vi "CDEx Redesign Controller for 3DoF Helicopter OnTheFly.vi"() -> ()   [LabVIEW 2009]
doc: "This example is derived from the Quanser (www.quanser.com) 3 DOF Helicopter academic challenge."
uses:
  <vilib>/addons/Control Design/_Model Construction/Model Creation.llb/Model Creation SubVI/cd_Create Symbolic State Space Model.vi
  <vilib>/Analysis/7linalg.llb/Create Special Real Matrix.vi
  3DHe_Global.vi
  <vilib>/addons/Control Design/_State Feedback Control/State Feedback Control.llb/State Feedback Control SubVis/cd_Linear Quadratic Regulator.vi
  <vilib>/Analysis/Matrix/Numeric/Conversions/Matrix To Array - RM.vi
  <vilib>/Analysis/NI_AALPro.lvlib
  <vilib>/addons/Control Design/_Model Construction/NI_LinSys_Model Creation.lvlib
  <vilib>/addons/Control Design/_State Feedback Control/NI_CD_State Feedback Control.lvlib
  <vilib>/Analysis/Matrix/NI_Matrix.lvlib
panel:
  in  "End":bool
  out "Tab Control":enum32{"Control Design: LQR"}(tab)
  in  "Diagonal of Q":dbl[](array[numeric])=[100.0, 100.0, 4000.0, 60.0, 100.0, 1500.0, 50.0, 10.0] format="%#.2g"
  out "Kep [V/deg]":dbl=-0.1888101782609241 format="%.2f"
  out "Ked [V/ deg sec^-1]":dbl=-0.148727007678325 format="%.2f"
  out "Kei [V/deg sec]":dbl=-0.07845852415328128 format="%.2f"
  out "Kpp [V/deg]":dbl=-0.40085841198215855 format="%.2f"
  out "Kpd [V/deg sec^-1]":dbl=-0.130295098559931 format="%.2f"
  out "Kpi":dbl format="%.2f"
  out "Ktp [deg/deg]":dbl=1.8918979439912578 format="%.2f"
  out "Ktd [deg/deg sec^-1]":dbl=2.9393753016474626 format="%.2f"
  out "Kti [deg/deg sec]":dbl=0.08753147368150993 format="%.2f"
  out "Optimal Gain (K)":dbl[][](array[numeric])=[[5.3810900382573665, 11.424464804866695, -21.613921777920005, 4.238719740944304, 3.7134103122560975, -33.580789896433664, 2.2360680469486356, -1.0000002670378931], [5.3810901226153085, -11.424464678116344, 21.613920933336832, 4.238719696720222, -3.71341030565997, 33.580789094931205, 2.2360678297883974, 1.000000202652513]] format="%.2f"
  in  "Design Method":u16(ring)=2 items=["manual", "stiff in elevation", "stiff in travel", "stiff in pitch", "minimize control"]
  in  "R":dbl[][](array[numeric])=[[5.0, 0.0], [0.0, 5.0]] format="%#.2g"
  in  "Q":dbl[][](array[numeric])=[[100.0, 0.0, 0.0, 0.0, 0.0, 0.0, 0.0, 0.0], [0.0, 100.0, 0.0, 0.0, 0.0, 0.0, 0.0, 0.0], [0.0, 0.0, 4000.0, 0.0, 0.0, 0.0, 0.0, 0.0], [0.0, 0.0, 0.0, 60.0, 0.0, 0.0, 0.0, 0.0], [0.0, 0.0, 0.0, 0.0, 100.0, 0.0, 0.0, 0.0], [0.0, 0.0, 0.0, 0.0, 0.0, 1500.0, 0.0, 0.0], [0.0, 0.0, 0.0, 0.0, 0.0, 0.0, 50.0, 0.0], [0.0, 0.0, 0.0, 0.0, 0.0, 0.0, 0.0, 10.0]] format="%#.2g"
  # "Derived Control Parameters\nfor PID Controllers from\nOptimal Gain"
  # "Control Design: LQR"
  # "Change the Design Method or the values in the Q and R matrices to verify the response in Simulation."
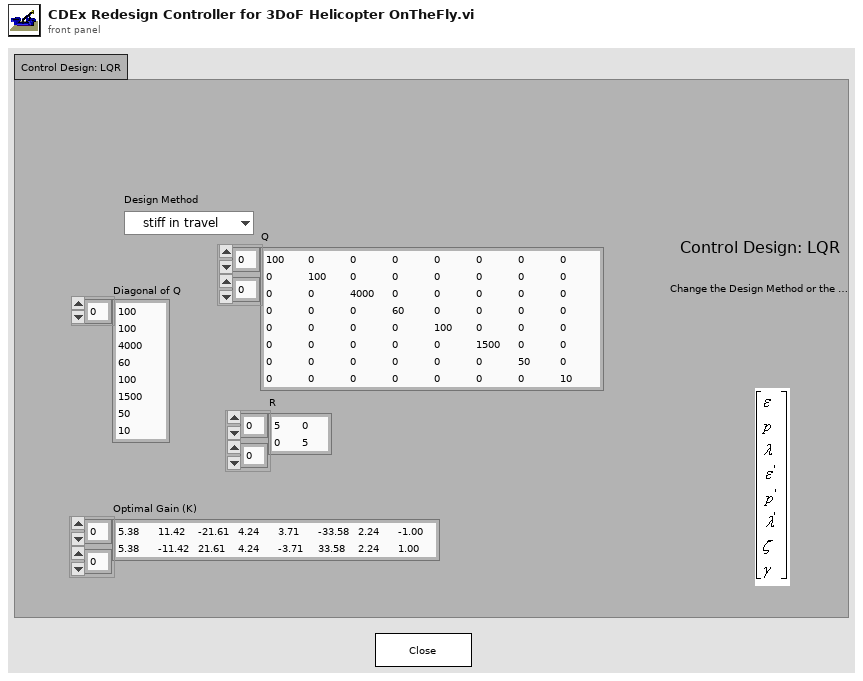
[diagram p1: front panel]
types:
  T1 = enum32{"Identity", "Diagonal", "Toepliz", "Vandermonde", "Companion"}
  T2 = typedef "NI_Matrix.lvlib/RealMatrix.ctl" = dbl[][]
  T3 = typedef "NI_LinSys_Model Typedefs.lvlib/CD State Space Model (MIMO).ctl" = cluster{"properties":T4, "A":dbl[][], "B":dbl[][], "C":dbl[][], "D":dbl[][], "StateNames":string[], "Transport Delay":dbl[][]}
  T4 = typedef "NI_LinSys_Model Typedefs.lvlib/CD General Elements.ctl" = cluster{"Model name":string, "Input names":string[], "Output names":string[], "Input Delays":dbl[], "Output Delays":dbl[], "Sampling Time":dbl, "Notes":string}
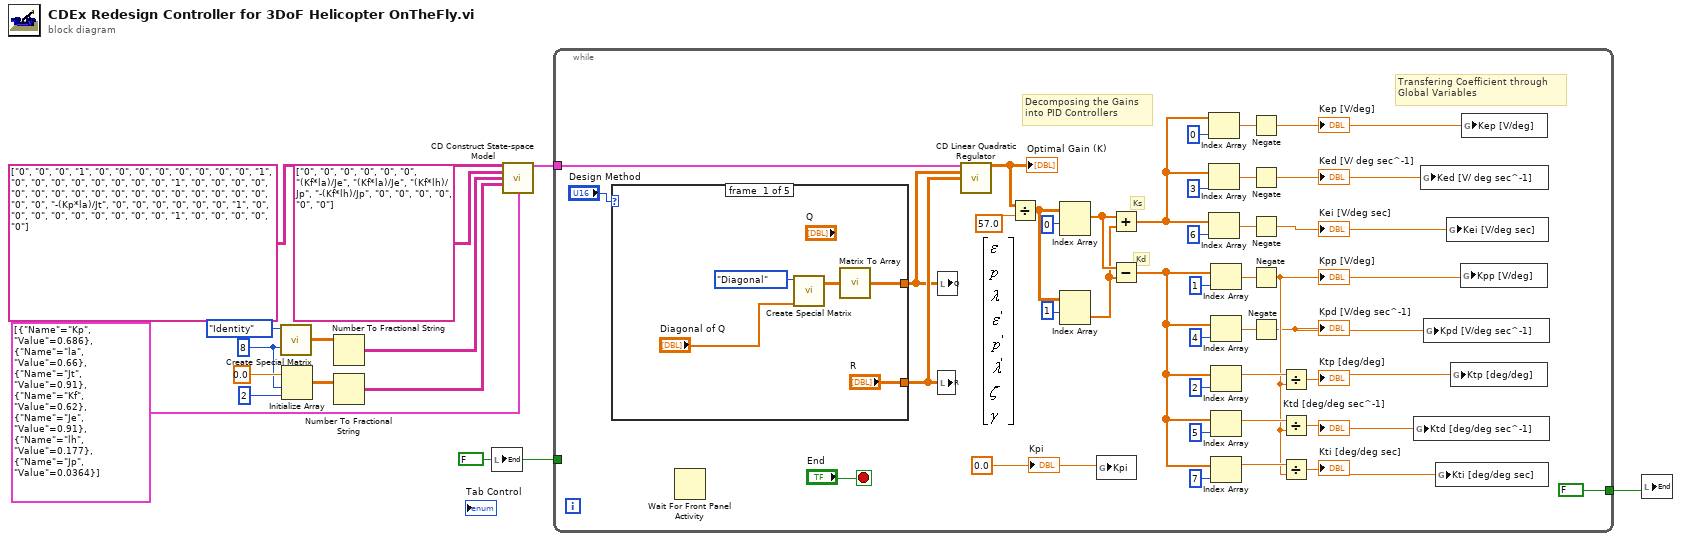
[diagram p0: block diagram]
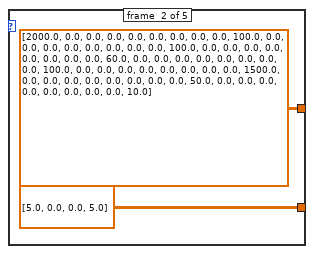
[diagram p2: hidden frame]
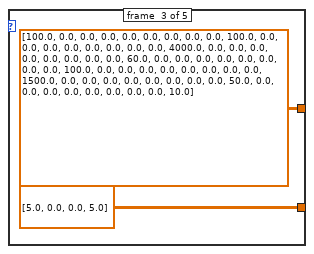
[diagram p3: hidden frame]
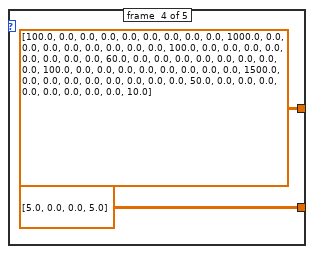
[diagram p4: hidden frame]
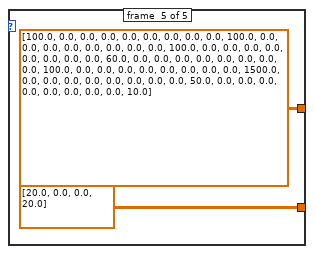
[diagram p5: hidden frame]
diagram:
  w2 = FALSE ("End")
  w9 = 8 ("matrix size")
  n1 = call-poly <vilib>:"Create Special Matrix.vi"("matrix type"=T1."Identity", "matrix size"=w9) -> ("Special Matrix"=w8:T2)  [unwired: 2 in, 2 out]
  n2 = Initialize Array(0.0 ("element"), w9, 2 ("dimension size")) -> (w12:dbl[][])
  n3 = Number To Fractional String(number=w8) -> (F-format string=w14:string[][])  [unwired: 3 out]
  n4 = Number To Fractional String(number=w12) -> (F-format string=w13:string[][])  [unwired: 3 out]
  n5 = local write "End"(w2) -> ()
  n6 = call-poly <vilib>:"CD Construct State-space Model.vi"("Symbolic A"=string[][] [["0", "0", "0", "1", "0", "0", "0", "0"], ["0", "0", "0", "0", "1", "0", "0", "0"], ["0", "0", "0", "0", "0", "1", "0", "0"], ["0", "0", "0", "0", "0", "0", "0", "0"], ["0", "0", "0", "0", "0", "0", "0", "0"], ["0", "-(Kp*la)/Jt", "0", "0", "0", "0", "0", "0"], ["1", "0", "0", "0", "0", "0", "0", "0"], ["0", "0", "1", "0", "0", "0", "0", "0"]] ("A"), "Symbolic B"=string[][] [["0", "0"], ["0", "0"], ["0", "0"], ["(Kf*la)/Je", "(Kf*la)/Je"], ["(Kf*lh)/Jp", "-(Kf*lh)/Jp"], ["0", "0"], ["0", "0"], ["0", "0"]] ("B"), "Symbolic C"=w14, "Symbolic D"=w13, "Variables"=cluster{"Name":string, "Value":dbl}[] [{"Name"="Kp", "Value"=0.686}, {"Name"="la", "Value"=0.66}, {"Name"="Jt", "Value"=0.91}, {"Name"="Kf", "Value"=0.62}, {"Name"="Je", "Value"=0.91}, {"Name"="lh", "Value"=0.177}, {"Name"="Jp", "Value"=0.0364}]) -> ("State Space Model"=w3:T3)  [unwired: 2 in, 8 out]
  n7 = while {
    tunnel: w3 -> [w54]
    tunnel: w2 -> [_]
    tunnel: [FALSE ("End")] -> w1
    stop <- "End" stop-if-true
    w26 = 0.0
    # "Transfering Coefficient through\nGlobal Variables"
    # "Decomposing the Gains\ninto PID Controllers"
    # "Kd"
    # "Ks"
    n8 = case shown="1" "Design Method" {
      tunnel: [w55 dbl[][] [[2000.0, 0.0, 0.0, 0.0, 0.0, 0.0, 0.0, 0.0], [0.0, 100.0, 0.0, 0.0, 0.0, 0.0, 0.0, 0.0], [0.0, 0.0, 100.0, 0.0, 0.0, 0.0, 0.0, 0.0], [0.0, 0.0, 0.0, 60.0, 0.0, 0.0, 0.0, 0.0], [0.0, 0.0, 0.0, 0.0, 100.0, 0.0, 0.0, 0.0], [0.0, 0.0, 0.0, 0.0, 0.0, 1500.0, 0.0, 0.0], [0.0, 0.0, 0.0, 0.0, 0.0, 0.0, 50.0, 0.0], [0.0, 0.0, 0.0, 0.0, 0.0, 0.0, 0.0, 10.0]] ("Q") dbl[][] [[100.0, 0.0, 0.0, 0.0, 0.0, 0.0, 0.0, 0.0], [0.0, 100.0, 0.0, 0.0, 0.0, 0.0, 0.0, 0.0], [0.0, 0.0, 4000.0, 0.0, 0.0, 0.0, 0.0, 0.0], [0.0, 0.0, 0.0, 60.0, 0.0, 0.0, 0.0, 0.0], [0.0, 0.0, 0.0, 0.0, 100.0, 0.0, 0.0, 0.0], [0.0, 0.0, 0.0, 0.0, 0.0, 1500.0, 0.0, 0.0], [0.0, 0.0, 0.0, 0.0, 0.0, 0.0, 50.0, 0.0], [0.0, 0.0, 0.0, 0.0, 0.0, 0.0, 0.0, 10.0]] ("Q") dbl[][] [[100.0, 0.0, 0.0, 0.0, 0.0, 0.0, 0.0, 0.0], [0.0, 1000.0, 0.0, 0.0, 0.0, 0.0, 0.0, 0.0], [0.0, 0.0, 100.0, 0.0, 0.0, 0.0, 0.0, 0.0], [0.0, 0.0, 0.0, 60.0, 0.0, 0.0, 0.0, 0.0], [0.0, 0.0, 0.0, 0.0, 100.0, 0.0, 0.0, 0.0], [0.0, 0.0, 0.0, 0.0, 0.0, 1500.0, 0.0, 0.0], [0.0, 0.0, 0.0, 0.0, 0.0, 0.0, 50.0, 0.0], [0.0, 0.0, 0.0, 0.0, 0.0, 0.0, 0.0, 10.0]] ("Q") dbl[][] [[100.0, 0.0, 0.0, 0.0, 0.0, 0.0, 0.0, 0.0], [0.0, 100.0, 0.0, 0.0, 0.0, 0.0, 0.0, 0.0], [0.0, 0.0, 100.0, 0.0, 0.0, 0.0, 0.0, 0.0], [0.0, 0.0, 0.0, 60.0, 0.0, 0.0, 0.0, 0.0], [0.0, 0.0, 0.0, 0.0, 100.0, 0.0, 0.0, 0.0], [0.0, 0.0, 0.0, 0.0, 0.0, 1500.0, 0.0, 0.0], [0.0, 0.0, 0.0, 0.0, 0.0, 0.0, 50.0, 0.0], [0.0, 0.0, 0.0, 0.0, 0.0, 0.0, 0.0, 10.0]] ("Q")] -> w27
      tunnel: ["R" dbl[][] [[5.0, 0.0], [0.0, 5.0]] ("R") dbl[][] [[5.0, 0.0], [0.0, 5.0]] ("R") dbl[][] [[5.0, 0.0], [0.0, 5.0]] ("R") dbl[][] [[20.0, 0.0], [0.0, 20.0]] ("R")] -> w28
      frame #0 {
        n9 = call-poly <vilib>:"Create Special Matrix.vi"("matrix type"=T1."Diagonal", "Input Vector1"="Diagonal of Q") -> ("Special Matrix"=w56:T2)  [unwired: 2 in, 2 out]
        n10 = call-poly <vilib>:"Matrix To Array.vi"("Real Matrix"=w56) -> ("Real 2D Array"=w55:dbl[][])
      }
      frame #1 {
      }
      frame #2 {
      }
      frame #3 {
      }
      frame #4 {
      }
    }
    n11 = Wait For Front Panel Activity() -> ()  [unwired: 4 out]
    n12 = local write "Q"(w27) -> ()
    n13 = local write "R"(w28) -> ()
    n14 = call-poly <vilib>:"CD Linear Quadratic Regulator.vi"("State-Space Model"=w54, "Q"=w27, "R"=w28) -> ("Optimal Gain (K)"=w17:dbl[][])  [unwired: 3 in, 9 out]
    "Optimal Gain (K)" <- w17
    n15 = Divide(x=w17, y=57.0) -> (x/y=w52:dbl[][])
    n16 = Index Array(array=w52, index (row)=0 ("disabled index (col)")) -> (element=w51:dbl[])  [unwired: 1 in]
    n17 = Index Array(array=w52, index (row)=1 ("disabled index (col)")) -> (element=w50:dbl[])  [unwired: 1 in]
    n18 = global write "3DHe_Global.vi" "Kpi"(w26) -> ()
    n19 = Add(x=w51, y=w50) -> (x+y=w41:dbl[])
    n20 = Subtract(x=w51, y=w50) -> (x-y=w33:dbl[])
    n21 = Index Array(array=w41, index=0) -> (element=w48:dbl)
    n22 = Index Array(array=w41, index=3) -> (element=w46:dbl)
    n23 = Index Array(array=w41, index=6) -> (element=w43:dbl)
    n24 = Index Array(array=w33, index=1) -> (element=w38:dbl)
    n25 = Index Array(array=w33, index=4) -> (element=w39:dbl)
    n26 = Index Array(array=w33, index=2) -> (element=w32:dbl)
    n27 = Index Array(array=w33, index=5) -> (element=w31:dbl)
    n28 = Index Array(array=w33, index=7) -> (element=w30:dbl)
    n29 = Negate(x=w48) -> (-x=w25:dbl)
    "Kep [V/deg]" <- w25
    n30 = Negate(x=w46) -> (-x=w24:dbl)
    "Ked [V/ deg sec^-1]" <- w24
    n31 = Negate(x=w43) -> (-x=w23:dbl)
    "Kei [V/deg sec]" <- w23
    n32 = Negate(x=w38) -> (-x=w22:dbl)
    "Kpp [V/deg]" <- w22
    n33 = Negate(x=w39) -> (-x=w18:dbl)
    "Kpd [V/deg sec^-1]" <- w18
    n34 = Divide(x=w32, y=w22) -> (x/y=w19:dbl)
    "Ktp [deg/deg]" <- w19
    n35 = Divide(x=w31, y=w22) -> (x/y=w20:dbl)
    "Ktd [deg/deg sec^-1]" <- w20
    n36 = Divide(x=w30, y=w22) -> (x/y=w21:dbl)
    "Kti [deg/deg sec]" <- w21
    n37 = global write "3DHe_Global.vi" "Ktd [deg/deg sec^-1]"(w20) -> ()
    n38 = global write "3DHe_Global.vi" "Ked [V/ deg sec^-1]"(w24) -> ()
    n39 = global write "3DHe_Global.vi" "Kpd [V/deg sec^-1]"(w18) -> ()
    n40 = global write "3DHe_Global.vi" "Kti [deg/deg sec]"(w21) -> ()
    n41 = global write "3DHe_Global.vi" "Kei [V/deg sec]"(w23) -> ()
    n42 = global write "3DHe_Global.vi" "Ktp [deg/deg]"(w19) -> ()
    n43 = global write "3DHe_Global.vi" "Kpp [V/deg]"(w22) -> ()
    n44 = global write "3DHe_Global.vi" "Kep [V/deg]"(w25) -> ()
    "Kpi" <- w26
  }
  n45 = local write "End"(w1) -> ()
